vi "select data range from peak.vi"(6 "Peak index":i32, 8 "Length":i32, 9 "Offset":dbl, 10 "Threshold":dbl format="%0.2f", 11 "In":dbl[][](array[numeric]) caption="input" format="%.2f") -> (3 "Out":dbl[][](array[numeric]))   [LabVIEW 2014]
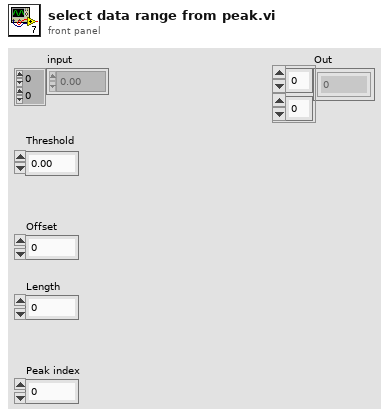
[diagram p1: front panel]
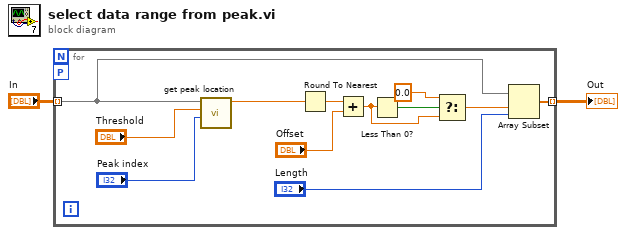
[diagram p0: block diagram]
diagram:
  n1 = for {
    tunnel: "In" -> [w10] mode=indexing
    tunnel: [w9] -> w1 mode=indexing
    workers-P: _ -> [_]
    n2 = call "get peak location.vi"("Peak index"="Peak index", "Threshold"="Threshold", "In"=w10) -> ("Numeric"=w14:dbl)  [unwired: 8 in]
    n3 = Round To Nearest(number=w14) -> (nearest integer value=w13:dbl)
    n4 = Add(x=w13, y="Offset") -> (x+y=w4:dbl)
    n5 = Less Than 0?(x=w4) -> (x < 0?=w6:bool)
    n6 = Select(t=0.0, s=w6, f=w4) -> (s? t:f=w3:dbl)
    n7 = Array Subset(array=w10, index=w3, length="Length") -> (w9:dbl[])
  }
  "Out" <- w1
